vi "ConvertFile.vi"(11 "String":string) -> (1 "Commands":string[](array[string]), 2 "cmd amd State":cluster{"Command":string, "End State":dbl[]}[](array[cluster]), 3 "flute dia (in)":dbl)   [LabVIEW 2023]
panel:
  out "Relative?":bool
  out "Absolute?":bool
  out "mm?":bool
  out "Inches?":bool
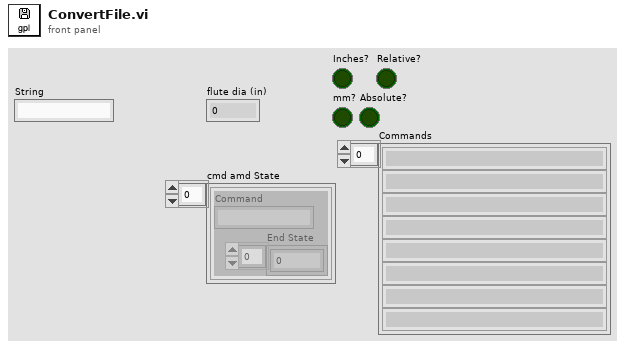
[diagram p1: front panel]
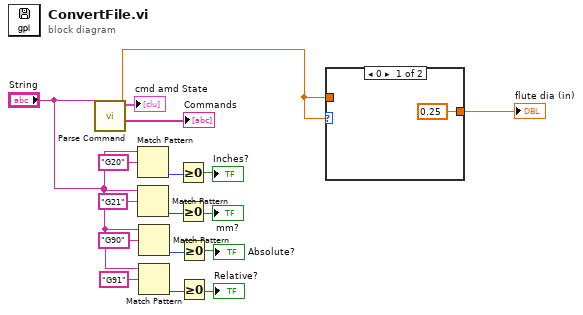
[diagram p0: block diagram]
diagram:
  n1 = call "Parse Command.vi"("text"="String") -> ("Commands"=→"Commands":string[], "flute dia (in)"=w1:dbl, "cmd amd State"=→"cmd amd State":cluster{"Command":string, "End State":dbl[]}[])  [unwired: 8 in]
  n2 = Match Pattern(string="String", regular expression="G20") -> (offset past match=w15:i32)  [unwired: 1 in, 3 out]
  n3 = Match Pattern(string="String", regular expression="G21") -> (offset past match=w13:i32)  [unwired: 1 in, 3 out]
  n4 = Match Pattern(string="String", regular expression="G90") -> (offset past match=w6:i32)  [unwired: 1 in, 3 out]
  n5 = Match Pattern(string="String", regular expression="G91") -> (offset past match=w8:i32)  [unwired: 1 in, 3 out]
  n6 = Greater Or Equal To 0?(x=w15) -> (x >= 0?=→"Inches?":bool)
  n7 = Greater Or Equal To 0?(x=w13) -> (x >= 0?=→"mm?":bool)
  n8 = Greater Or Equal To 0?(x=w6) -> (x >= 0?=→"Absolute?":bool)
  n9 = Greater Or Equal To 0?(x=w8) -> (x >= 0?=→"Relative?":bool)
  n10 = case shown="0" w1 {
    tunnel: [0.25 ("flute dia (in)") w19] -> w2
    tunnel: w1 -> [_ w19]
    frame 0 {
    }
    frame Default {
    }
  }
  "flute dia (in)" <- w2
